vi "Get The Channel Data Type and Length.vi"(8 "error in (no error)":errorcluster, 9 "channel name":string, 10 "group name":string, 11 "tdms file":refnum<k34>) -> (0 "error out":errorcluster, 1 "dup channel name":string, 2 "dup group name":string, 3 "dup tdms file":refnum<k34>, 4 "channel length":i32, 6 "data type":i32)   [LabVIEW 2023]
doc: "Get the data type and channel length of a specified channel."
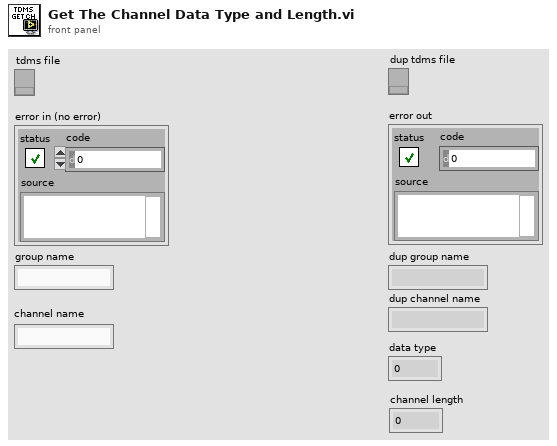
[diagram p1: front panel]
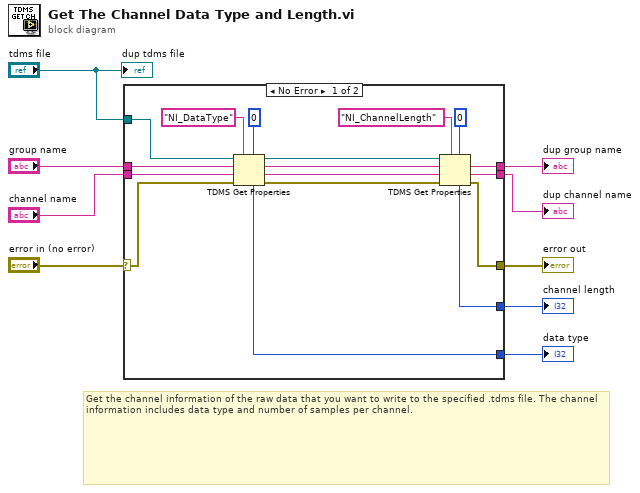
[diagram p0: block diagram]
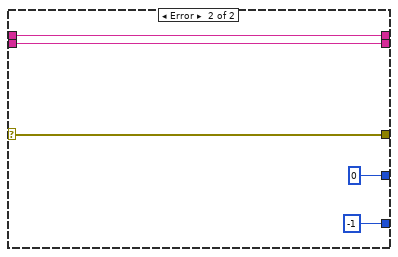
[diagram p2: hidden frame]
diagram:
  # "Get the channel information of the raw data that you want to write to the specified .tdms file. The channel information includes data type and number of samples per channel."
  n1 = case shown="No Error" "error in (no error)" {
    selector: "error in (no error)" -> [w14 w29]
    tunnel: [w23 w29] -> w9
    tunnel: "tdms file" -> [w22 _]
    tunnel: "channel name" -> [w21 w30]
    tunnel: "group name" -> [w20 w31]
    tunnel: [w19 -1] -> w6
    tunnel: [w17 0] -> w5
    tunnel: [w16 w31] -> w4
    tunnel: [w15 w30] -> w3
    frame No Error {
      n2 = TDMS Get Properties(5:0, 7:"NI_DataType", 8:w14, 9:w21, 10:w20, 11:w22) -> (0:w10:errorcluster, 1:w11:string, 2:w12:string, 3:w13:refnum<k34>, 4:w19:i32)  [unwired: 1 out]
      n3 = TDMS Get Properties(5:0, 7:"NI_ChannelLength" ("property name"), 8:w10, 9:w11, 10:w12, 11:w13) -> (0:w23:errorcluster, 1:w15:string, 2:w16:string, 4:w17:i32)  [unwired: 2 out]
    }
    frame Error {
    }
  }
  "error out" <- w9
  "data type" <- w6
  "channel length" <- w5
  "dup group name" <- w4
  "dup channel name" <- w3
  "dup tdms file" <- "tdms file"
